vi "refresh parameters.vi"(8 "error in (no error)":errorcluster, 9 "runtime.Fitting.FIT_A.Fitting parameters":T1, 10 "cluster":T2, 11 "LineCCD in":refnum<class "LineCCD.lvclass">) -> (0 "error out":errorcluster, 3 "LineCCD out":refnum<class "LineCCD.lvclass">)   [LabVIEW 2012, in "LineCCD.lvclass"]
uses:
  LineCCD.lvclass
  fitting parameters.ctl
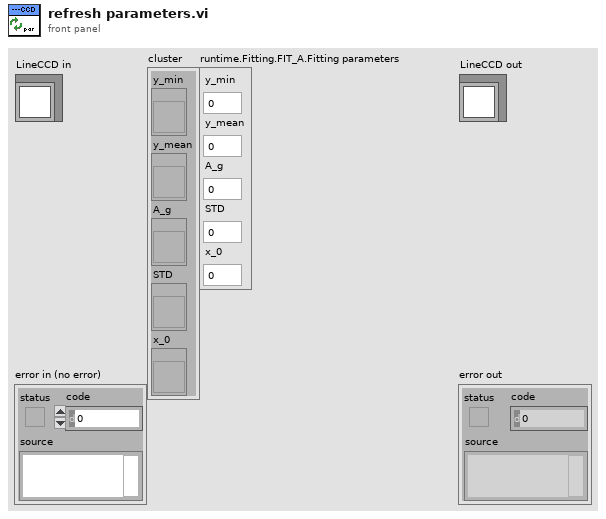
[diagram p1: front panel]
types:
  T1 = typedef "LineCCD.lvclass/fitting parameters.ctl" = cluster{"y_min":dbl, "y_mean":dbl, "A_g":dbl, "STD":dbl, "x_0":dbl}
  T2 = cluster{"y_min":refnum<vi>, "y_mean":refnum<vi>, "A_g":refnum<vi>, "STD":refnum<vi>, "x_0":refnum<vi>}
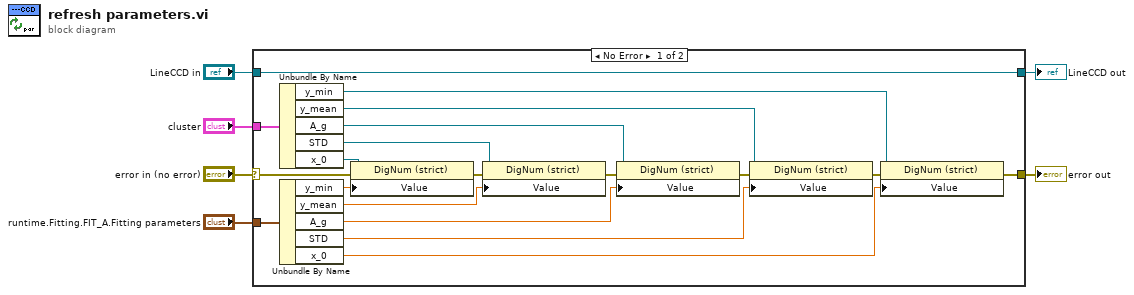
[diagram p0: block diagram]
diagram:
  n1 = case shown="No Error" "error in (no error)" {
    selector: "error in (no error)" -> [w21 w27]
    tunnel: [w20 w27] -> w5
    tunnel: [w13 w26] -> w3
    tunnel: "LineCCD in" -> [w13 w26]
    tunnel: "cluster" -> [w19 _]
    tunnel: "runtime.Fitting.FIT_A.Fitting parameters" -> [w12 _]
    frame No Error {
      n2 = Unbundle By Name(w19) -> ("y_min"=w14:refnum<vi>, "y_mean"=w15:refnum<vi>, "A_g"=w16:refnum<vi>, "STD"=w17:refnum<vi>, "x_0"=w18:refnum<vi>)
      n3 = Unbundle By Name(w12) -> ("y_min"=w11:dbl, "y_mean"=w10:dbl, "A_g"=w9:dbl, "STD"=w8:dbl, "x_0"=w7:dbl)
      n4 = property class="DigNum (strict)"(reference=w18, error in=w21, "Value"=w11) -> (error out=w22:errorcluster)  [unwired: 1 out]
      n5 = property class="DigNum (strict)"(reference=w17, error in=w22, "Value"=w10) -> (error out=w23:errorcluster)  [unwired: 1 out]
      n6 = property class="DigNum (strict)"(reference=w16, error in=w23, "Value"=w9) -> (error out=w24:errorcluster)  [unwired: 1 out]
      n7 = property class="DigNum (strict)"(reference=w15, error in=w24, "Value"=w8) -> (error out=w25:errorcluster)  [unwired: 1 out]
      n8 = property class="DigNum (strict)"(reference=w14, error in=w25, "Value"=w7) -> (error out=w20:errorcluster)  [unwired: 1 out]
    }
    frame Error {
    }
  }
  "error out" <- w5
  "LineCCD out" <- w3
